vi "Set Variable.vi"(8 "error in (no error)":errorcluster, 9 "Value":dbl, 10 "Name":string, 11 "Sequence in":refnum<class "Sequence.lvclass">) -> (0 "error out":errorcluster, 2 "Not Found":bool, 3 "Sequence out":refnum<class "Sequence.lvclass">)   [LabVIEW 2020, in "VolatusSeq.lvlib" / "Sequence.lvclass"]
uses:
  Sequence.lvclass
  Sequence.lvclass/Sequence.ctl
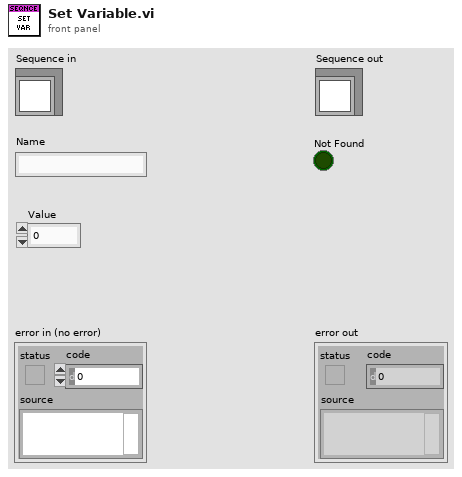
[diagram p1: front panel]
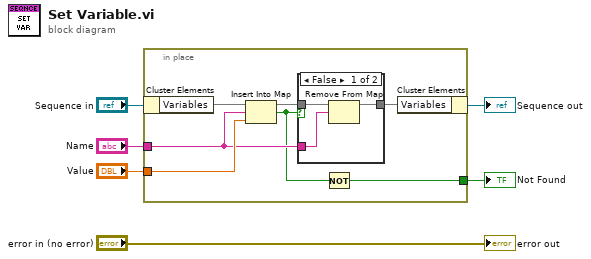
[diagram p0: block diagram]
diagram:
  n1 = in-place {
    in-place-border: "Name" -> [w9]
    in-place-border: "Value" -> [w12]
    in-place-border: [w7] -> w2
    n2 = in-place-cluster #1("Sequence in") -> ("Variables"=w13:map{string, dbl})
    n3 = Insert Into Map(map in=w13, key=w9, value=w12) -> (map out=w11:map{string, dbl}, key already included?=w8:bool)  [unwired: 1 out]
    n4 = case shown="False" w8 {
      tunnel: w11 -> [w16 w17]
      tunnel: [w14 w17] -> w10
      tunnel: w9 -> [w15 _]
      frame False {
        n5 = Remove From Map(10:w15, 11:w16) -> (3:w14:map{string, dbl})  [unwired: 2 out]
      }
      frame True {
      }
    }
    n6 = Not(x=w8) -> (.not. x?=w7:bool)
    n7 = in-place-cluster #1("Variables"=w10) -> (→"Sequence out":refnum<class "Sequence.lvclass">)
  }
  "Not Found" <- w2
  "error out" <- "error in (no error)"
